vi "Cheby approx_2Darray_DV.vi"(4 "Y-array":dbl[](array[numeric]), 6 "X-array":dbl[](array[numeric]), 7 "x and f(x)":string="0.47166\t0.04369\n0.48675\t0.04561\n0.50232\t0.0476\n0.5184\t0.04965\n0.53498\t0.05177\n0.5521\t0.05396\n0.56976\t0.05621\n0.588\t0.0589\n0.60681\t0.06196\n0.62622\t0.06512\n0.64626\t0.06837\n0.66694\t0.07174\n0.68828\t0.07518\n0.7103\t0.07865\n0.73303\t0.08223\n0.75648\t0.08593\n0.78068\t0.08975\n0.80566\t0.09466\n0.83144\t0.10012\n0.85804\t0.10576\n0.8855\t0.11158\n0.91383\t0.11759\n0.94307\t0.12379\n0.97325\t0.13101\n1.00439\t0.13851\n1.03652\t0.14625\n1.06969\t0.15425\n1.10391\t0.16251\n1.13923\t0.17103\n1.17568\t0.18593\n1.2133\t0.20556\n1.25212\t0.22582\n1.29219\t0.24675\n1.33353\t0.26835\n1.3762\t0.29198\n1.42023\t0.31887\n1.46567\t0.34662\n1.51257\t0.37527\n1.56097\t0.40486\n1.61091\t0.4354\n1.66245\t0.46693\n1.71565\t0.50366\n1.77054\t0.5425\n1.82719\t0.5826\n1.88565\t0.62401\n1.94599\t0.66675\n2.00825\t0.70939\n2.07251\t0.75065\n2.13882\t0.79326\n2.20725\t0.83725\n2.27788\t0.88267\n2.35076\t0.92957\n2.42598\t0.98463\n2.5036\t1.05538\n2.5837\t1.12843\n2.66637\t1.20384\n2.75169\t1.28171\n2.83973\t1.3621\n2.93059\t1.44636\n3.02436\t1.53862\n3.12113\t1.63388\n3.22099\t1.73223\n3.32405\t1.83377\n3.43041\t1.93861\n3.54017\t2.04685\n3.65344\t2.1586\n3.77033\t2.27398\n3.89097\t2.3931\n4.01547\t2.53674\n4.14395\t2.69895\n4.27654\t2.86642\n4.41337\t3.03932\n4.55458\t3.21431\n4.70031\t3.39354\n4.8507\t3.57859\n5.0059\t3.76964\n5.16607\t3.96689\n5.33137\t4.13732\n5.50195\t4.29297\n5.67799\t4.45366\n5.85967\t4.61958\n6.04715\t4.79936\n6.24064\t5.00776\n6.44032\t5.22292\n6.64638\t5.44506\n6.85904\t5.63666\n7.0785\t5.7907\n7.30499\t5.94975\n7.53872\t6.119\n7.77993\t6.35913\n8.02886\t6.60705\n8.28575\t6.86211\n8.55086\t6.95953\n8.82445\t7.06011\n9.1068\t7.16396\n9.39819\t7.27118\n9.69889\t7.38188\n10.0092\t7.44894\n10.3295\t7.49568\n10.66\t7.54569\n11.0011\t7.60164\n11.353\t7.65941\n11.7163\t7.71342\n12.0912\t7.64668\n12.4781\t7.57777\n12.8773\t7.50663\n13.2893\t7.43318\n13.7145\t7.36236\n14.1533\t7.30161\n14.6062\t7.23888\n15.0735\t7.17412\n15.5558\t7.10726\n16.0536\t7.04646\n16.5672\t6.99619\n17.0973\t6.94428\n17.6443\t6.8907\n18.2089\t6.83537\n18.7915\t6.80319\n19.3928\t6.79324\n20.0133\t6.78296\n20.6536\t6.77236\n21.3144\t6.7614\n21.9964\t6.8054\n22.7002\t6.91834\n23.4265\t7.03494\n24.1761\t7.15532\n24.9496\t7.27962\n25.7479\t7.45801\n26.5718\t7.889\n27.422\t8.33397\n28.2994\t8.79339\n29.2048\t9.26772\n30.1393\t9.7666\n31.1036\t10.2936\n32.0988\t10.8378\n33.1259\t11.3996\n34.1858\t11.9797\n35.2796\t12.5228\n36.4084\t13.0316\n37.5733\t13.557\n38.7755\t14.0994\n40.0162\t14.6594\n41.2965\t15.2376\n42.6179\t15.7758\n43.9815\t16.1744\n45.3887\t16.5858\n46.841\t17.0106\n48.3397\t17.4492\n49.8864\t17.765\n51.4826\t18.0492\n53.1298\t18.3427\n54.8298\t18.6457\n56.5841\t18.949\n58.3946\t18.9931\n60.263\t19.0387\n62.1912\t19.0858\n64.181\t19.1344\n66.2346\t19.1845\n68.3538\t19.0548\n70.5409\t18.9111\n72.7979\t18.7628\n75.1272\t18.6097\n77.531\t18.4162\n80.0117\t18.183\n82.5717\t17.9422\n85.2137\t17.6936\n87.9402\t17.4369\n90.754\t17.1637\n93.6577\t16.8762\n96.6544\t16.5793\n99.747\t16.2728\n102.939\t15.9563\n106.232\t15.6484\n109.631\t15.3755\n113.139\t15.0936\n116.759\t14.8027\n120.495\t14.5022\n124.35\t14.1959\n128.329\t13.9348\n132.435\t13.6653\n136.672\t13.387\n141.045\t13.0997\n145.558\t12.8156\n150.216\t12.5313\n155.022\t12.2378\n159.982\t11.9348\n165.101\t11.6219\n170.383\t11.4173\n175.835\t11.3293\n181.461\t11.2384\n187.267\t11.1446\n193.259\t11.0478\n199.442\t10.9478\n205.824\t10.9239\n212.409\t10.9096\n219.206\t10.8949\n226.219\t10.8797\n233.458\t10.8641\n240.927\t11.0173\n248.636\t11.1932", 8 "order":u32=14, 9 "end":dbl=7.0 format="%.2f", 10 "start":dbl format="%.2f", 11 "number of points":u32=56) -> (1 "best y-fit":dbl[](array[numeric]), 2 "x arry out":dbl[](array[numeric]), 3 "Tn coeffs":dbl[](array[numeric])=[-1.4885517808010453, -0.4725618709636064, 0.4630200814142276, 0.6700741417747852, -0.15642761844645178, -0.10776354749193232, -0.019394804254517988, 0.02480718958930428, 0.011086294796594199, -0.02220834303954161, 0.014194437393199913, 0.00192073719401433, -0.013619305726609358, 0.012299938256651008] format="%.2f")   [LabVIEW 2021]
uses:
  Cheby polynomial/Cheby 2D array prep_XY arrays.vi
panel:
  out "XY Graph":cluster{dbl[], dbl[]}[](graph)
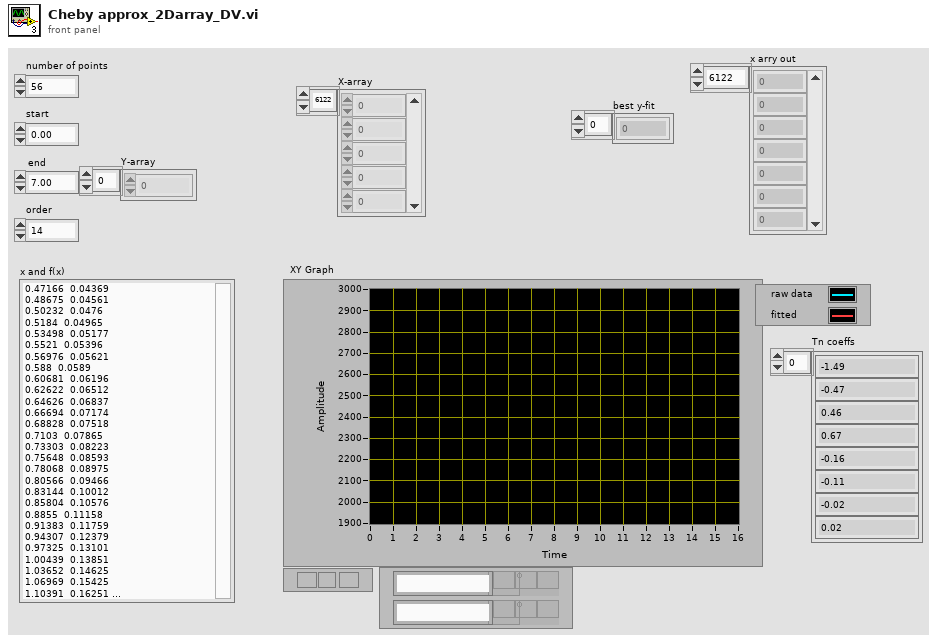
[diagram p1: front panel]
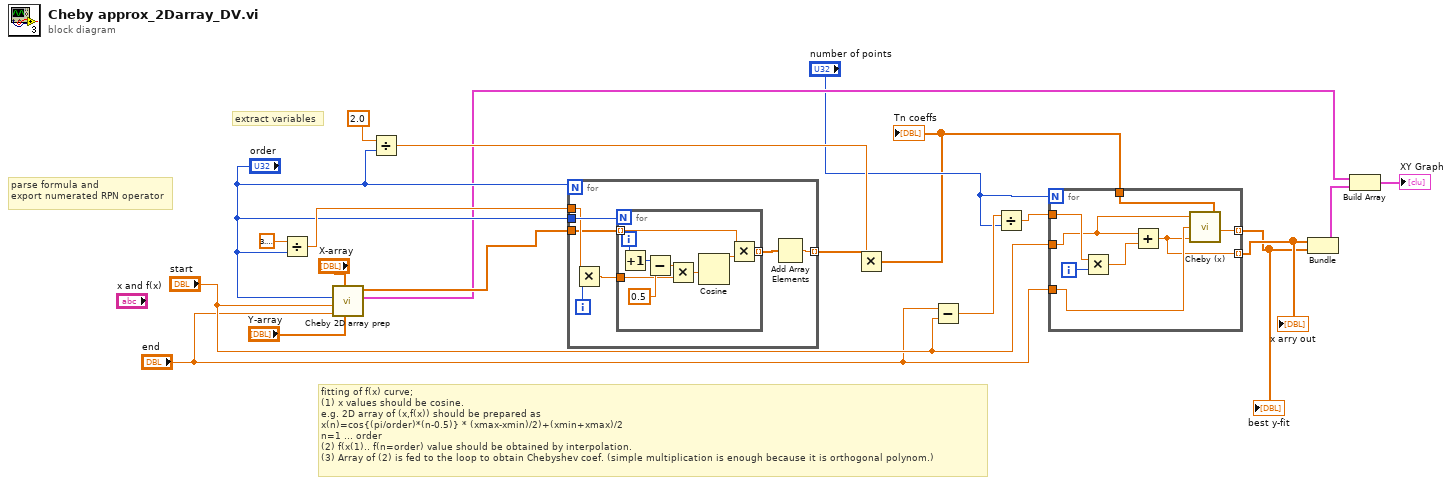
[diagram p0: block diagram]
diagram:
  # "extract variables"
  # "fitting of f(x) curve;\n(1) x values should be cosine.\ne.g. 2D array of (x,f(x)) should be prepared as \nx(n)=cos{(pi/order)*(n-0.5)} * (xmax-xmin)/2)+(xmin+xmax)/2 \nn=1 ... order\n(2) f(x(1).. f(n=order) value should be obtained by interpolation.\n(3) Array of (2) is fed to the loop to obtain Chebyshev coef. (simple multiplication is enough because it is orthogonal polynom.)"
  # "parse formula and\nexport numerated RPN operator"
  n1 = Divide(x=3.141592653589793, y="order") -> (x/y=w16:dbl)
  n2 = call-poly "Cheby 2D array prep.vi"("Y-array"="Y-array", "X-array"="X-array", "end"="end", "start"="start", "order"="order") -> ("original curve"=w12:cluster{dbl[], dbl[]}, "values"=w14:dbl[])  [unwired: 4 in]
  n3 = Divide(x=2.0, y="order") -> (x/y=w18:dbl)
  n4 = for {
    N: "order" -> [_]
    tunnel: "order" -> [w27]
    tunnel: w16 -> [w26]
    tunnel: w14 -> [w24]
    tunnel: [w22] -> w19 mode=indexing
    i -> [w21]
    n5 = Multiply(x=w26, y=w21) -> (x*y=w25:dbl)
    n6 = for {
      N: w27 -> [_]
      tunnel: w25 -> [w28]
      tunnel: w24 -> [w35] mode=indexing
      tunnel: [w34] -> w23 mode=indexing
      i -> [w33]
      n7 = Increment(x=w33) -> (x+1=w29:i32)
      n8 = Subtract(x=w29, y=0.5) -> (x-y=w31:dbl)
      n9 = Multiply(x=w31, y=w28) -> (x*y=w30:dbl)
      n10 = Cosine(x=w30) -> (cos(x)=w36:dbl)
      n11 = Multiply(x=w35, y=w36) -> (x*y=w34:dbl)
    }
    n12 = Add Array Elements(numeric array=w23) -> (sum=w22:dbl)
  }
  n13 = Multiply(x=w18, y=w19) -> (x*y=w6:dbl[])
  "Tn coeffs" <- w6
  n14 = Subtract(x="end", y="start") -> (x-y=w11:dbl)
  n15 = Divide(x=w11, y="number of points") -> (x/y=w8:dbl)
  n16 = for {
    N: "number of points" -> [_]
    tunnel: "start" -> [w41]
    tunnel: w8 -> [w44]
    tunnel: "end" -> [w40]
    tunnel: w6 -> [w39]
    tunnel: [w38] -> w4 mode=indexing
    tunnel: [w37] -> w5 mode=indexing
    i -> [w43]
    n17 = Multiply(x=w44, y=w43) -> (x*y=w42:dbl)
    n18 = Add(x=w41, y=w42) -> (x+y=w37:dbl)
    n19 = call "Cheby (x).vi"("Tn coeffs"=w39, "x"=w37, "end"=w40, "start"=w41) -> ("f(x)"=w38:dbl)
  }
  "x arry out" <- w5
  "best y-fit" <- w4
  n20 = Bundle(w5, w4) -> (w3:cluster{dbl[], dbl[]})  [unwired: 1 in]
  n21 = Build Array(w12, w3) -> (→"XY Graph":cluster{dbl[], dbl[]}[])
